vi "SubVI_Prescan Limit.vi"(8 "Input trace 2D array":dbl[][](array[numeric]), 11 "Limit":T1) -> (0 "Output Limit Cluster":cluster{"xi used":dbl[], "yi":dbl[]}, 1 "limit 1D array":dbl[](array[numeric]), 2 "frequency 1D array":dbl[](array[numeric]), 3 "Output limit 2D array":dbl[][](array[numeric]))   [LabVIEW 2016]
doc: "this SubVI load limit line onto the XY graph"
uses:
  Limit.ctl
  <vilib>/gmath/NI_Gmath.lvlib
panel:
  out "Number of points":i32
  out "XY Graph":cluster{"xi used":dbl[], "yi":dbl[]}(graph)
  out "Trace Frequency":dbl[](array[numeric])
  out "Trace amplitude":dbl[](array[numeric])
  out "Limit Frequency":dbl[](array[numeric])
  out "Limit Value":dbl[](array[numeric])
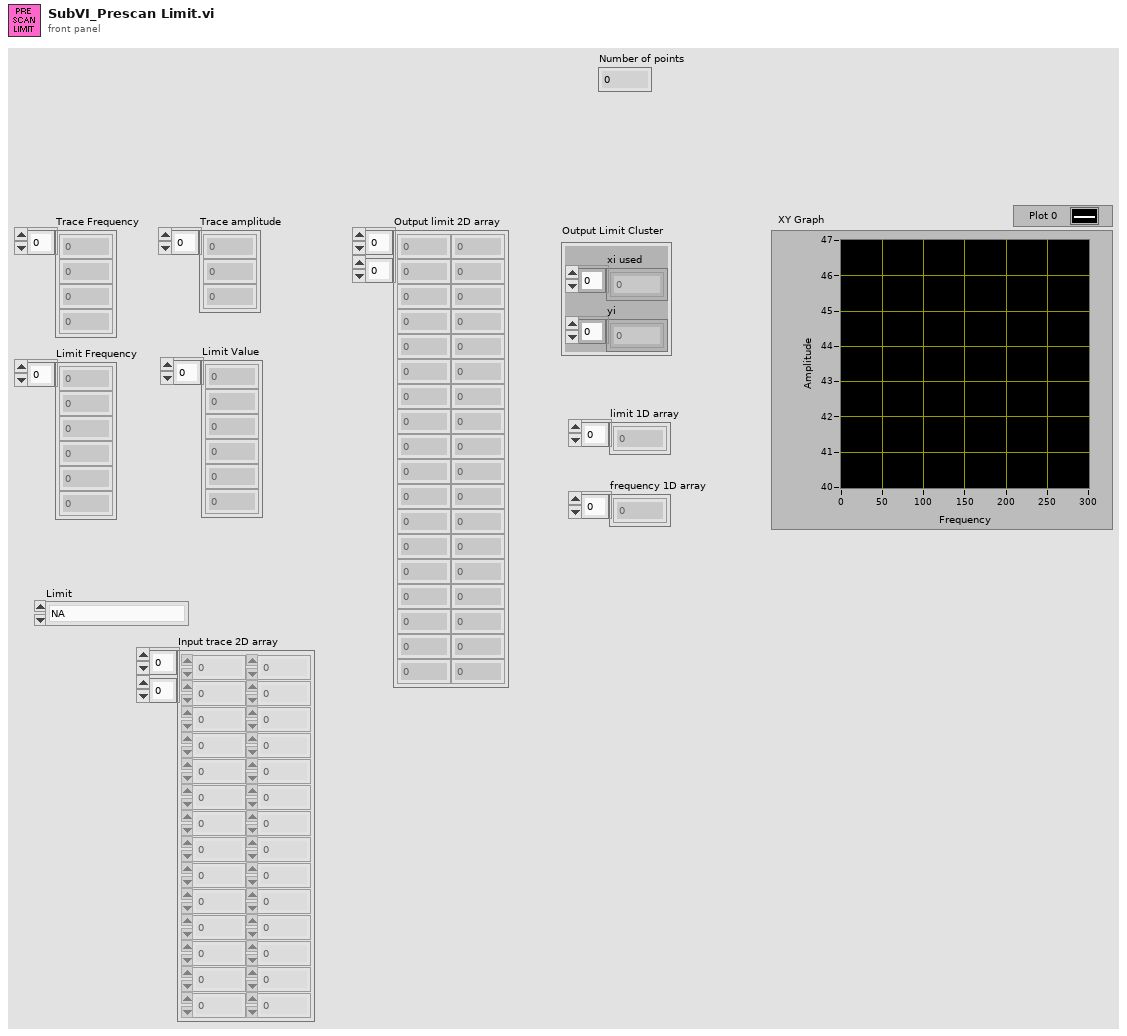
[diagram p1: front panel]
types:
  T1 = typedef "Limit.ctl" = enum16{"NA", "CISPR32 ClassB @ 3m"}
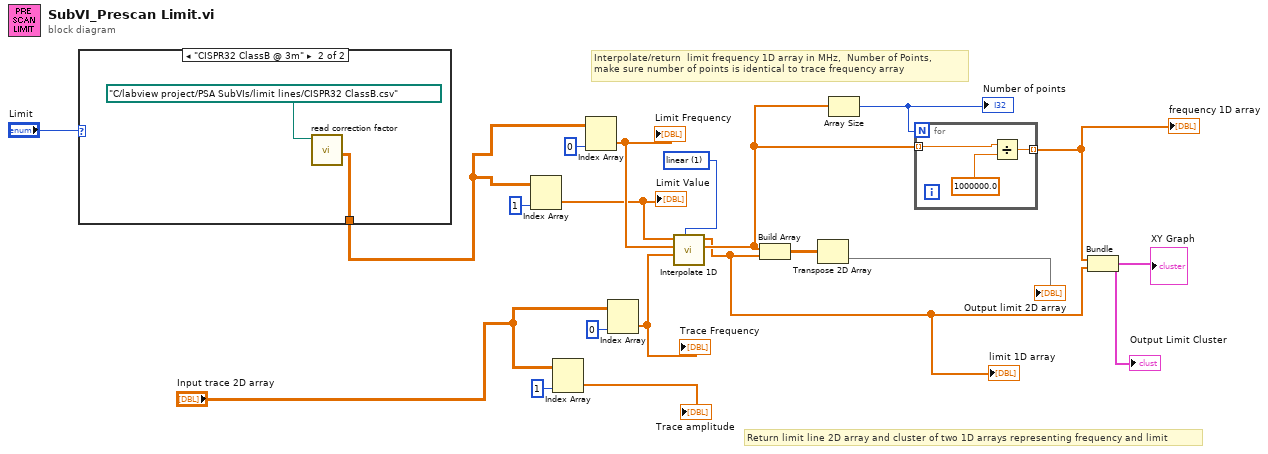
[diagram p0: block diagram]
diagram:
  w8 = 1 items=["nearest", "linear", "spline", "cubic Hermite", "Lagrange"] ("method")
  # "Interpolate/return  limit frequency 1D array in MHz,  Number of Points,\nmake sure number of points is identical to trace frequency array"
  # "Return limit line 2D array and cluster of two 1D arrays representing frequency and limit"
  n1 = case shown="\"CISPR32 ClassB @ 3m\"" "Limit" {
    tunnel: [_ w20] -> w3
    frame "NA", Default {
    }
    frame "CISPR32 ClassB @ 3m" {
      n2 = call "read correction factor.vi"("Path"=path "C:/labview project/PSA SubVIs/limit lines/CISPR32 ClassB.csv") -> ("Output Array"=w20:dbl[][])  [unwired: 7 in, 3 out]
    }
  }
  n3 = Index Array(array=w3, index (col)=1 ("disabled index (col)")) -> (element=w12:dbl[])  [unwired: 1 in]
  "Limit Value" <- w12
  n4 = Index Array(array="Input trace 2D array", index (col)=1 ("disabled index (col)")) -> (element=→"Trace amplitude":dbl[])  [unwired: 1 in]
  n5 = Index Array(array=w3, index (col)=0 ("disabled index (col)")) -> (element=w13:dbl[])  [unwired: 1 in]
  "Limit Frequency" <- w13
  n6 = Index Array(array="Input trace 2D array", index (col)=0 ("disabled index (col)")) -> (element=w14:dbl[])  [unwired: 1 in]
  "Trace Frequency" <- w14
  n7 = call <vilib>:"Interpolate 1D.vi"("method"=w8, "xi"=w14, "X"=w13, "Y"=w12) -> ("xi used"=w6:dbl[], "yi"=w1:dbl[])  [unwired: 5 in, 1 out]
  "limit 1D array" <- w1
  n8 = Build Array(w6, w1) -> (w10:dbl[][])
  n9 = Transpose 2D Array(2D array=w10) -> (transposed array=→"Output limit 2D array":dbl[][])
  n10 = Array Size(array=w6) -> (size(s)=w7:i32)
  "Number of points" <- w7
  n11 = for {
    N: w7 -> [_]
    tunnel: w6 -> [w23] mode=indexing
    tunnel: [w22] -> w5 mode=indexing
    n12 = Divide(x=w23, y=1000000.0) -> (x/y=w22:dbl)
  }
  "frequency 1D array" <- w5
  n13 = Bundle(w5, "yi"=w1) -> (→"XY Graph" →"Output Limit Cluster":cluster{dbl[], "yi":dbl[]})  [unwired: 1 in]
